vi "busy_wait.vi"(7 "caller":refnum<vi>, 8 "error in (no error)":errorcluster, 11 "configuration":T1={"dialog_text"="", "boolean_text_1"="", "boolean_text_2"="", "boolean_text_3"="", "inner_color"=16711680, "outer_color"=6618880, "wait_s"=nan, "error_status"=FALSE, "error_source"="", "error_details"="", "string []"=[], "custom_entry"=FALSE}) -> (0 "error out":errorcluster, 3 "failed/cancelled?":bool)   [LabVIEW 2015, in "lv-dialog-interfaces.lvlib"]
uses:
  lv-dialog-interfaces.lvlib
  lv-dialog/api/v1/public/_controls/configuration.ctl
  _controls/dialog_type.ctl
  _controls/hmi_references.ctl
  lv-dialog/api/v1/public/_controls/dialog_selection.ctl
  <vilib>/ptbypt/NI_PtbyPt.lvlib
  lv-dialog/api/v1/v1.lvlib
panel:
  out "dialog":string
  out "busy":u16(knob) scale=0.0..20.0
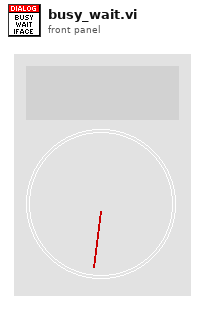
[diagram p1: front panel]
types:
  T1 = typedef "lv-dialog.lvlib/v1.lvlib/configuration.ctl" = cluster{"dialog_text":string, "boolean_text_1":string, "boolean_text_2":string, "boolean_text_3":string, "inner_color":u32, "outer_color":u32, "wait_s":dbl, "error_status":bool, "error_source":string, "error_details":string, "string []":string[], "custom_entry":bool}
  T2 = typedef "lv-dialog-interfaces.lvlib/dialog_type.ctl" = enum16{"null", "one_button", "two_button", "three_button", "confirmation", "busy_wait", "error", "busy_wait_embed", "combo_box", "data_entry_string", "data_entry_numeric"}
  T3 = typedef "lv-dialog-interfaces.lvlib/hmi_references.ctl" = cluster{"vi_reference":refnum<vi>, "caller":refnum<vi>, "dialog":refnum<vi>, "button_1":refnum<vi>, "button_2":refnum<vi>, "button_3":refnum<vi>, "busy":refnum<vi>, "error_glyph":refnum<vi>, "error_source":refnum<vi>, "error_text":refnum<vi>, "combo_box":refnum<vi>}
  T4 = typedef "lv-dialog.lvlib/v1.lvlib/dialog_selection.ctl" = enum16{"null", "panel_closed", "button_1", "button_2", "button_3", "cancelled"}
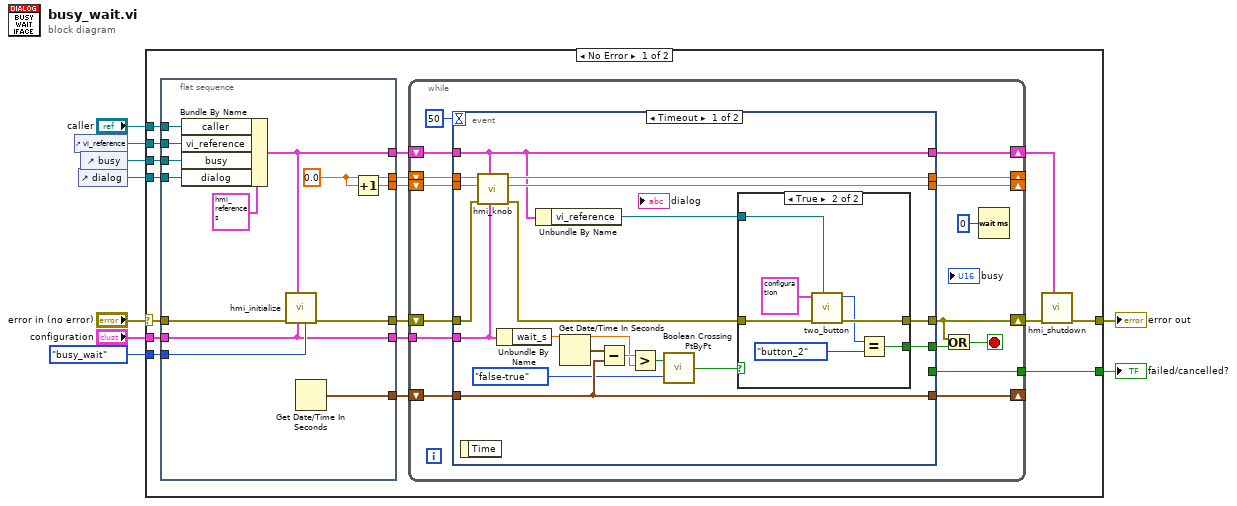
[diagram p0: block diagram]
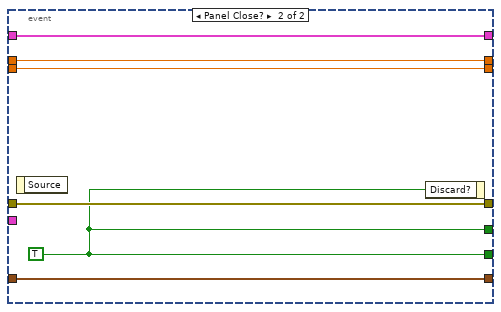
[diagram p3: hidden frame]
diagram:
  n1 = control-ref of="vi_reference"() -> (w3:refnum<vi>)
  n2 = control-ref of="dialog"() -> (w1:refnum<vi>)
  n3 = control-ref of="busy"() -> (w2:refnum<vi>)
  n4 = case shown="No Error" "error in (no error)" {
    selector: "error in (no error)" -> [w26 w88]
    tunnel: [w25 _] -> w8
    tunnel: "caller" -> [w24 _]
    tunnel: "configuration" -> [w23 _]
    tunnel: dialog_type."busy_wait" ("dialog_type") -> [w22 _]
    tunnel: [w20 w88] -> w4
    tunnel: w3 -> [w12 _]
    tunnel: w2 -> [w11 _]
    tunnel: w1 -> [w10 _]
    frame No Error {
      n5 = flat-sequence {
        tunnel: [w39] -> w19
        tunnel: [w38] -> w18
        tunnel: [w31] -> w17
        tunnel: w26 -> [w37]
        tunnel: [w33] -> w16
        tunnel: [w32] -> w15
        tunnel: w23 -> [w30]
        tunnel: [w30] -> w14
        tunnel: w24 -> [w35]
        tunnel: w22 -> [w34]
        tunnel: w12 -> [w29]
        tunnel: w11 -> [w28]
        tunnel: w10 -> [w27]
        frame #0 {
          w32 = 0.0
          n6 = Bundle By Name(cluster=T3 {"vi_reference"=refnum, "caller"=refnum, "dialog"=refnum, "button_1"=refnum, "button_2"=refnum, "button_3"=refnum, "busy"=refnum, "error_glyph"=refnum, "error_source"=refnum, "error_text"=refnum, "combo_box"=refnum} ("references"), "caller"=w35, "vi_reference"=w29, "busy"=w28, "dialog"=w27) -> (w31:T3)
          n7 = call "hmi_initialize.vi"("dialog_type"=w34, "configuration"=w30, "references"=w31, "error in (no error)"=w37) -> ("error out"=w33:errorcluster)  [unwired: 7 in]
          n8 = Get Date/Time In Seconds() -> (seconds since 1Jan1904=w38:timestamp)
          n9 = Increment(x=w32) -> (x+1=w39:dbl)
        }
      }
      n10 = while {
        shift-right: [w55] -> _
        shift-left: w15 -> [w52]
        shift-right: [w54] -> _
        shift-left: w19 -> [w53]
        shift-right: [w41] -> w21
        shift-left: w16 -> [w51]
        shift-right: [w47] -> _
        shift-left: w18 -> [w48]
        tunnel: [w46] -> w25
        tunnel: w14 -> [w45]
        shift-right: [w40] -> w13
        shift-left: w17 -> [w44]
        stop <- w42 stop-if-true
        n11 = event shown="[0] Timeout" {
          selector: _ -> [_ _]
          dyn-events: _ -> [_ _]
          timeout: 50 -> [_ _]
          tunnel: [w63 w86] -> w55
          tunnel: [w64 w85] -> w54
          tunnel: w53 -> [w62 w85]
          tunnel: w52 -> [w61 w86]
          tunnel: w51 -> [w73 w87]
          tunnel: [w66 w87] -> w41
          tunnel: [w56 w84] -> w43
          tunnel: w48 -> [w71 w83]
          tunnel: [w71 w83] -> w47
          tunnel: [w56 w84] -> w46
          tunnel: w45 -> [w59 _]
          tunnel: w44 -> [w58 w82]
          tunnel: [w58 w82] -> w40
          event Timeout {
            n12 = event-data() -> ()  [unwired: 1 in, 1 out]
            n13 = call "hmi_knob.vi"("configuration"=w59, "hmi_references"=w58, "error in (no error)"=w73, "value_2 in"=w62, "value_1 in"=w61) -> ("error out"=w67:errorcluster, "value_2 out"=w64:dbl, "value_1 out"=w63:dbl)  [unwired: 4 in]
            n14 = Unbundle By Name(w59) -> ("wait_s"=w60:dbl)
            n15 = Unbundle By Name(w58) -> ("vi_reference"=w57:refnum<vi>)
            n16 = Get Date/Time In Seconds() -> (seconds since 1Jan1904=w72:timestamp)
            n17 = Subtract(x=w72, y=w71) -> (x-y=w70:dbl)
            n18 = Greater?(x=w70, y=w60) -> (0:w69:bool)
            n19 = call <vilib>:"Boolean Crossing PtByPt.vi"("direction"=enum16{"either", "false-true", "true-false"}."false-true", "input"=w69) -> ("crossing"=w65:bool)  [unwired: 1 in]
            n20 = case shown="True" w65 {
              tunnel: w67 -> [w74 w78]
              tunnel: [w74 w77] -> w66
              tunnel: [_ w80] -> w56
              tunnel: w57 -> [_ w75]
              frame False {
              }
              frame True {
                n21 = call "two_button.vi"("callee"=w75, "error in (no error)"=w78, "configuration"=T1 {"dialog_text"="Waiting process has not completed.", "boolean_text_1"="Wait", "boolean_text_2"="Continue", "boolean_text_3"="", "inner_color"=16711680, "outer_color"=6618880, "wait_s"=nan, "error_status"=FALSE, "error_source"="", "error_details"="", "string []"=[], "custom_entry"=FALSE} ("configuration 2")) -> ("error out"=w77:errorcluster, "dialog_selection"=w76:T4)  [unwired: 7 in]
                n22 = Equal?(x=w76, y=dialog_selection."button_2" ("x")) -> (x = y?=w80:bool)
              }
            }
          }
          event Panel Close? {
            w84 = TRUE
            n23 = event-data() -> ()  [unwired: 1 in, 1 out]
            n24 = event-data("Discard?"=w84) -> ()  [unwired: 1 in, 1 out]
          }
        }
        n25 = Or(x=w41, y=w43) -> (x .or. y?=w42:bool)
        n26 = Wait (ms)(milliseconds to wait=u32 0) -> ()  [unwired: 1 out]
      }
      n27 = call "hmi_shutdown.vi"("references"=w13, "error in (no error)"=w21) -> ("error out"=w20:errorcluster)  [unwired: 9 in]
    }
    frame Error {
    }
  }
  "error out" <- w4
  "failed/cancelled?" <- w8
